vi "Read Configuration File.vi"(8 "error in (no error)":errorcluster, 11 "Instrument.FrameworkTemplate":refnum<class "Instrument.FrameworkTemplate.lvclass">) -> (0 "error out":errorcluster, 3 "Instrument.FrameworkTemplate out":refnum<class "Instrument.FrameworkTemplate.lvclass">)   [LabVIEW 2019, in "Instrument.FrameworkTemplate.lvclass"]
uses:
  Instrument.FrameworkTemplate.lvclass
  C:/Program Files (x86)/National Instruments/LabVIEW 2019/user.lib/LevyLab/Levylab Instruments/SMOs/Instrument/Instrument.lvclass
  <userlib>/LevyLab/Levylab Instruments/SMOs/Instrument/Instrument.lvclass/Instrument.ctl
  Instrument.FrameworkTemplate.lvclass/Instrument.FrameworkTemplate.ctl
  <userlib>/LevyLab/Levylab Instruments/SMOs/Configuration/Configuration.lvclass
  <userlib>/LevyLab/Levylab Instruments/SMOs/Instrument/Instrument.lvclass
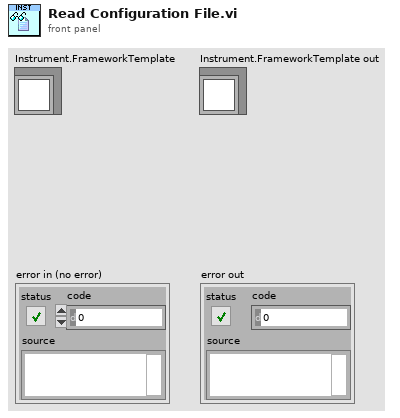
[diagram p1: front panel]
types:
  T1 = typedef "Instrument.FrameworkTemplate.lvclass/Instrument.FrameworkTemplate.Configuration--Cluster.ctl" = cluster{"Example Setting 1":dbl, "Example Setting 2":dbl, "Example Setting 3":string}
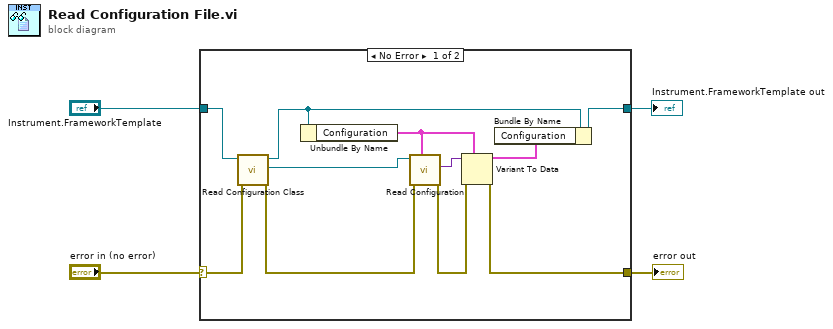
[diagram p0: block diagram]
diagram:
  n1 = case shown="No Error" "error in (no error)" {
    selector: "error in (no error)" -> [w9 w17]
    tunnel: "Instrument.FrameworkTemplate" -> [w12 w16]
    tunnel: [w7 w16] -> w3
    tunnel: [w10 w17] -> w2
    frame No Error {
      n2 = call <userlib>:"Read Configuration Class.vi"("error in (no error)"=w9, "Instrument in"=w12) -> ("error out"=w13:errorcluster, "Configuration"=w14:refnum<class "Configuration.lvclass">, "Instrument out"=w6:refnum<class "Instrument.FrameworkTemplate.lvclass">)  [unwired: 7 in]
      n3 = Unbundle By Name(w6) -> ("Configuration"=w8:T1)
      n4 = call <userlib>:"Read Configuration.vi"("INI Fomatted Cluster Type"=w8, "error in (no error)"=w13, "Configuration in"=w14) -> ("error out"=w15:errorcluster, "Configuration"=w5:variant)  [unwired: 6 in, 1 out]
      n5 = Variant To Data(error in=w15, type=w8, Variant=w5) -> (data=w11:T1, error out=w10:errorcluster)
      n6 = Bundle By Name(cluster=w6, "Configuration"=w11) -> (w7:refnum<class "Instrument.FrameworkTemplate.lvclass">)
    }
    frame Error {
    }
  }
  "Instrument.FrameworkTemplate out" <- w3
  "error out" <- w2
